vi "MotionProfilingLogging.vi"(11 "Main Talon":T1={"DeviceStatus"={"status"=FALSE, "code"=0, "source"=""}, "Type"=enum."PWM", "PWM"={"PWM Channel"=enum."Invalid", "DeadBand"={"Name"="", "maxPositivePwm"=0, "minPositivePwm"=0, "centerPwm"=0, "maxNegativePwm"=0, "minNegativePwm"=0, "angularRange"=0}}, "CAN"={"Device Number"=0, "SetOutput VI Ref"=variant(enum8{"Percent VBus", "Current", "Speed", "Position", "Voltage"} enum."Percent VBus"), "GetOutput VI Ref"=variant(refnum<k1> refnum), "Enable VI Ref"=variant(dbl 12.0), "Disable VI Ref"=variant(enum8{"Percent VBus", "Speed", "Position", "Slave", "Unchanged / Invalid", "Voltage Compensation", "Current", "Motion Profile"} enum."Percent VBus"), "Data"=variant}, "Invert"=FALSE, "DIO PWM"={"PWM \"Enable\" Channel"=enum."Invalid", "DIOChannel"=enum."Invalid", "PWM Rate"=0.0}}) -> ()   [LabVIEW 2018]
uses:
  <vilib>/Rock Robotics/WPI/MotorControl/WPI_MotorControlDeviceRef.ctl
  <vilib>/Rock Robotics/WPI/MotorControl/WPI_MotorControlType.ctl
  <vilib>/Rock Robotics/SystemInterfaces/DIO/FPGA_DIOPWMChannel.ctl
  <vilib>/Rock Robotics/WPI/PWM/WPI_PWMDeadband.ctl
  <vilib>/Rock Robotics/SystemInterfaces/DIO/FPGA_DIOChannel.ctl
  <userlib>/836-Library/System/TDMS_V2/Support/TDMS_DevRef.ctl
  <userlib>/836-Library/System/TDMS_V2/Support/Logging_Settings.ctl
  <userlib>/836-Library/System/TDMS_V2/Support/Group_FIFO_Config.ctl
  <userlib>/836-Library/System/TDMS_V2/Support/Channel_FIFO_Config.ctl
  Subsystems/Drive/driveShifterEnum.ctl
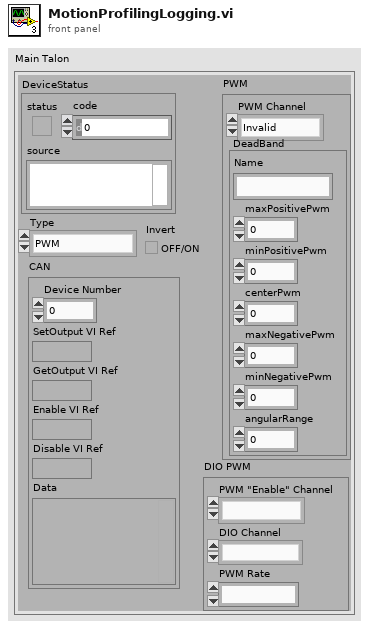
[diagram p1: front panel]
types:
  T1 = typedef "WPI_MotorControlDeviceRef.ctl" = cluster{"DeviceStatus":errorcluster, "Type":T2, "PWM":cluster{"PWM Channel":T3, "DeadBand":T4}, "CAN":cluster{"Device Number":u8, "SetOutput VI Ref":variant, "GetOutput VI Ref":variant, "Enable VI Ref":variant, "Disable VI Ref":variant, "Data":variant}, "Invert":bool, "DIO PWM":cluster{"PWM \"Enable\" Channel":T3, "DIOChannel":T5, "PWM Rate":dbl}}
  T2 = typedef "WPI_MotorControlType.ctl" = enum16{"PWM", "CAN", "DIO PWM"}
  T3 = typedef "FPGA_DIOPWMChannel.ctl" = enum8{"PWM 0", "PWM 1", "PWM 2", "PWM 3", "PWM 4", "PWM 5", "PWM 6", "PWM 7", "PWM 8", "PWM 9", "PWM MXP 0", "PWM MXP 1", "PWM MXP 2", "PWM MXP 3", "PWM MXP 4", "PWM MXP 5", "PWM MXP 6", "PWM MXP 7", "PWM MXP 8", "PWM MXP 9", "Invalid"}
  T4 = typedef "WPI_PWMDeadband.ctl" = cluster{"Name":string, "maxPositivePwm":i32, "minPositivePwm":i32, "centerPwm":i32, "maxNegativePwm":i32, "minNegativePwm":i32, "angularRange":u16}
  T5 = typedef "FPGA_DIOChannel.ctl" = enum8{"DIO 0", "DIO 1", "DIO 2", "DIO 3", "DIO 4", "DIO 5", "DIO 6", "DIO 7", "DIO 8", "DIO 9", "DIO MXP 0", "DIO MXP 1", "DIO MXP 2", "DIO MXP 3", "DIO MXP 4", "DIO MXP 5", "DIO MXP 6", "DIO MXP 7", "DIO MXP 8", "DIO MXP 9", "DIO MXP 10", "DIO MXP 11", "DIO MXP 12", "DIO MXP 13", "DIO MXP 14", "DIO MXP 15", "SPI Port CS1", "SPI Port CS2", "SPI Port CS3", "SPI Port MISO", "SPI Port MOSI", "Invalid"}
  T6 = enum16{"Inches -> Sensor Units", "Sensor Units -> Inches"}
  T7 = typedef "driveShifterEnum.ctl" = enum16{"Low", "High"}
  T8 = cluster{"Top Buffer Remaining":i32, "Top Buffer Count":i32, "Bottom Buffer Count":i32, "Has Underrun?":bool, "Is Underrun?":bool, "Active Point Valid?":bool, "Is Last?":bool, "Profile Slot Select 0":i32, "Output Enable":i32, "Time Duration (ms)":i32, "Profile Slot Select 1":i32}
  T9 = typedef "TDMS_DevRef.ctl" = cluster{"Name":string, "File Ref":refnum<k34>, "Start Time":timestamp, "Logging Settings":T10, "Group FIFO Config":T11[], "Data To Write":refnum<data-value>, "semaphore":T13, "Ref Time Reset":refnum<k4>}
  T10 = typedef "Logging_Settings.ctl" = cluster{"Data Grab Period":dbl, "File Write Period":dbl, "Max Stored Size":dbl, "Burst Size":dbl}
  T11 = typedef "Group_FIFO_Config.ctl" = cluster{"Group":string, "Channels":T12[], "Channel Names":string[]}
  T12 = typedef "Channel_FIFO_Config.ctl" = cluster{"Channel":string, "FIFO":refnum<k33>}
  T13 = typedef "Semaphore RefNum" = refnum<k1>
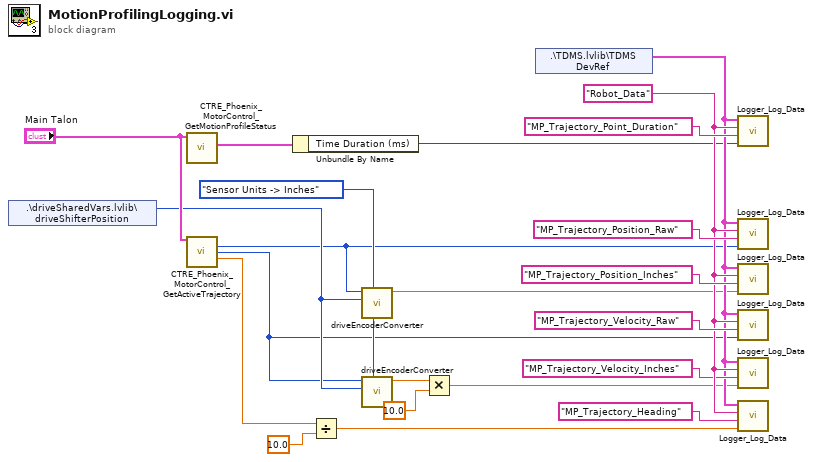
[diagram p0: block diagram]
diagram:
  w10 = T6."Sensor Units -> Inches" ("Conversion Direction")
  w15 = "Robot_Data" ("Group")
  n1 = shared-variable ".\\driveSharedVars.lvlib\\driveShifterPosition"() -> (w11:T7)  [unwired: 1 in, 1 out]
  n2 = call <vilib>:"CTRE_Phoenix_MotorControl_GetMotionProfileStatus.vi"("PhoenixMotorControlDevRef"="Main Talon") -> ("Motion Profile Status"=w21:T8)  [unwired: 8 in, 2 out]
  n3 = call <vilib>:"CTRE_Phoenix_MotorControl_GetActiveTrajectory.vi"("PhoenixMotorControlDevRef"="Main Talon") -> ("Position (Sensor Units)"=w9:i32, "Velocity (Sensor Units per 100 ms)"=w7:i32, "Heading"=w3:dbl)  [unwired: 10 in, 2 out]
  n4 = Unbundle By Name(w21) -> ("Time Duration (ms)"=w12:i32)
  n5 = Divide(x=w3, y=10.0) -> (x/y=w1:dbl)
  n6 = call "driveEncoderConverter.vi"("Conversion Direction"=w10, "Gear Setting"=w11, "Input"=w9) -> ("Output"=w8:dbl)  [unwired: 8 in]
  n7 = call "driveEncoderConverter.vi"("Conversion Direction"=w10, "Gear Setting"=w11, "Input"=w7) -> ("Output"=w6:dbl)  [unwired: 8 in]
  n8 = Multiply(x=w6, y=10.0) -> (x*y=w4:dbl)
  n9 = shared-variable ".\\TDMS.lvlib\\TDMS DevRef"() -> (w13:T9)  [unwired: 1 in, 1 out]
  n10 = call <userlib>:"Logger_Log_Data.vi"("Data"=w12, "Channel"="MP_Trajectory_Point_Duration", "Group"=w15, "TDMS DevRef"=w13) -> ()  [unwired: 7 in, 1 out]
  n11 = call <userlib>:"Logger_Log_Data.vi"("Data"=w9, "Channel"="MP_Trajectory_Position_Raw", "Group"=w15, "TDMS DevRef"=w13) -> ()  [unwired: 7 in, 1 out]
  n12 = call <userlib>:"Logger_Log_Data.vi"("Data"=w8, "Channel"="MP_Trajectory_Position_Inches", "Group"=w15, "TDMS DevRef"=w13) -> ()  [unwired: 7 in, 1 out]
  n13 = call <userlib>:"Logger_Log_Data.vi"("Data"=w7, "Channel"="MP_Trajectory_Velocity_Raw", "Group"=w15, "TDMS DevRef"=w13) -> ()  [unwired: 7 in, 1 out]
  n14 = call <userlib>:"Logger_Log_Data.vi"("Data"=w4, "Channel"="MP_Trajectory_Velocity_Inches", "Group"=w15, "TDMS DevRef"=w13) -> ()  [unwired: 7 in, 1 out]
  n15 = call <userlib>:"Logger_Log_Data.vi"("Data"=w1, "Channel"="MP_Trajectory_Heading", "Group"=w15, "TDMS DevRef"=w13) -> ()  [unwired: 7 in, 1 out]
